vi "Control.vi"() -> ()   [LabVIEW 2012]
uses:
  <vilib>/express/express analysis/Spectral/Block/exnSpectralBlock spectral measurements peak poly.vi
  <vilib>/express/express analysis/Spectral/Block/exnSpectralBlock spectral measurements peak DDT.vi
  <vilib>/express/express analysis/Spectral/XNode/ExpressSpectralMeasurementsBlockNode.xnode
  <vilib>/Analysis/NI_AALPro.lvlib
panel:
  out "Waveform Graph":dynamicdata(graph)
  out "GrabO 5":dbl[](array[numeric])
  out "GrabO 4":dbl[](array[numeric])
  out "In Range?":bool[](array[boolean])
  out "Entrada":dbl[](array[numeric])
  out "GrabO 3":dbl[](array[numeric])
  out "GrabO 2":dbl[](array[numeric])
  out "GrabO":dbl[](array[numeric])
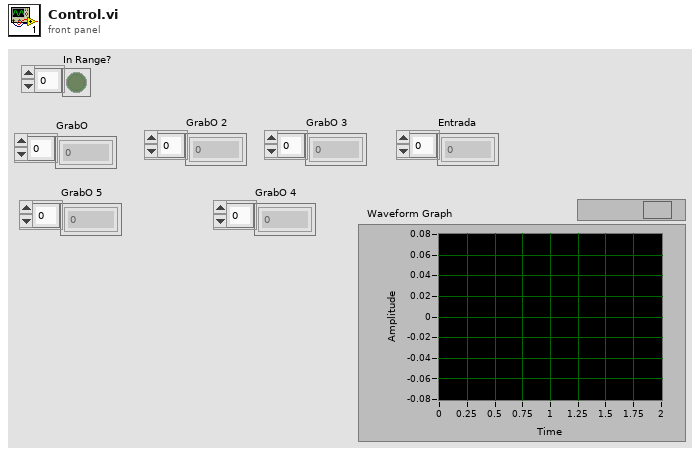
[diagram p1: front panel]
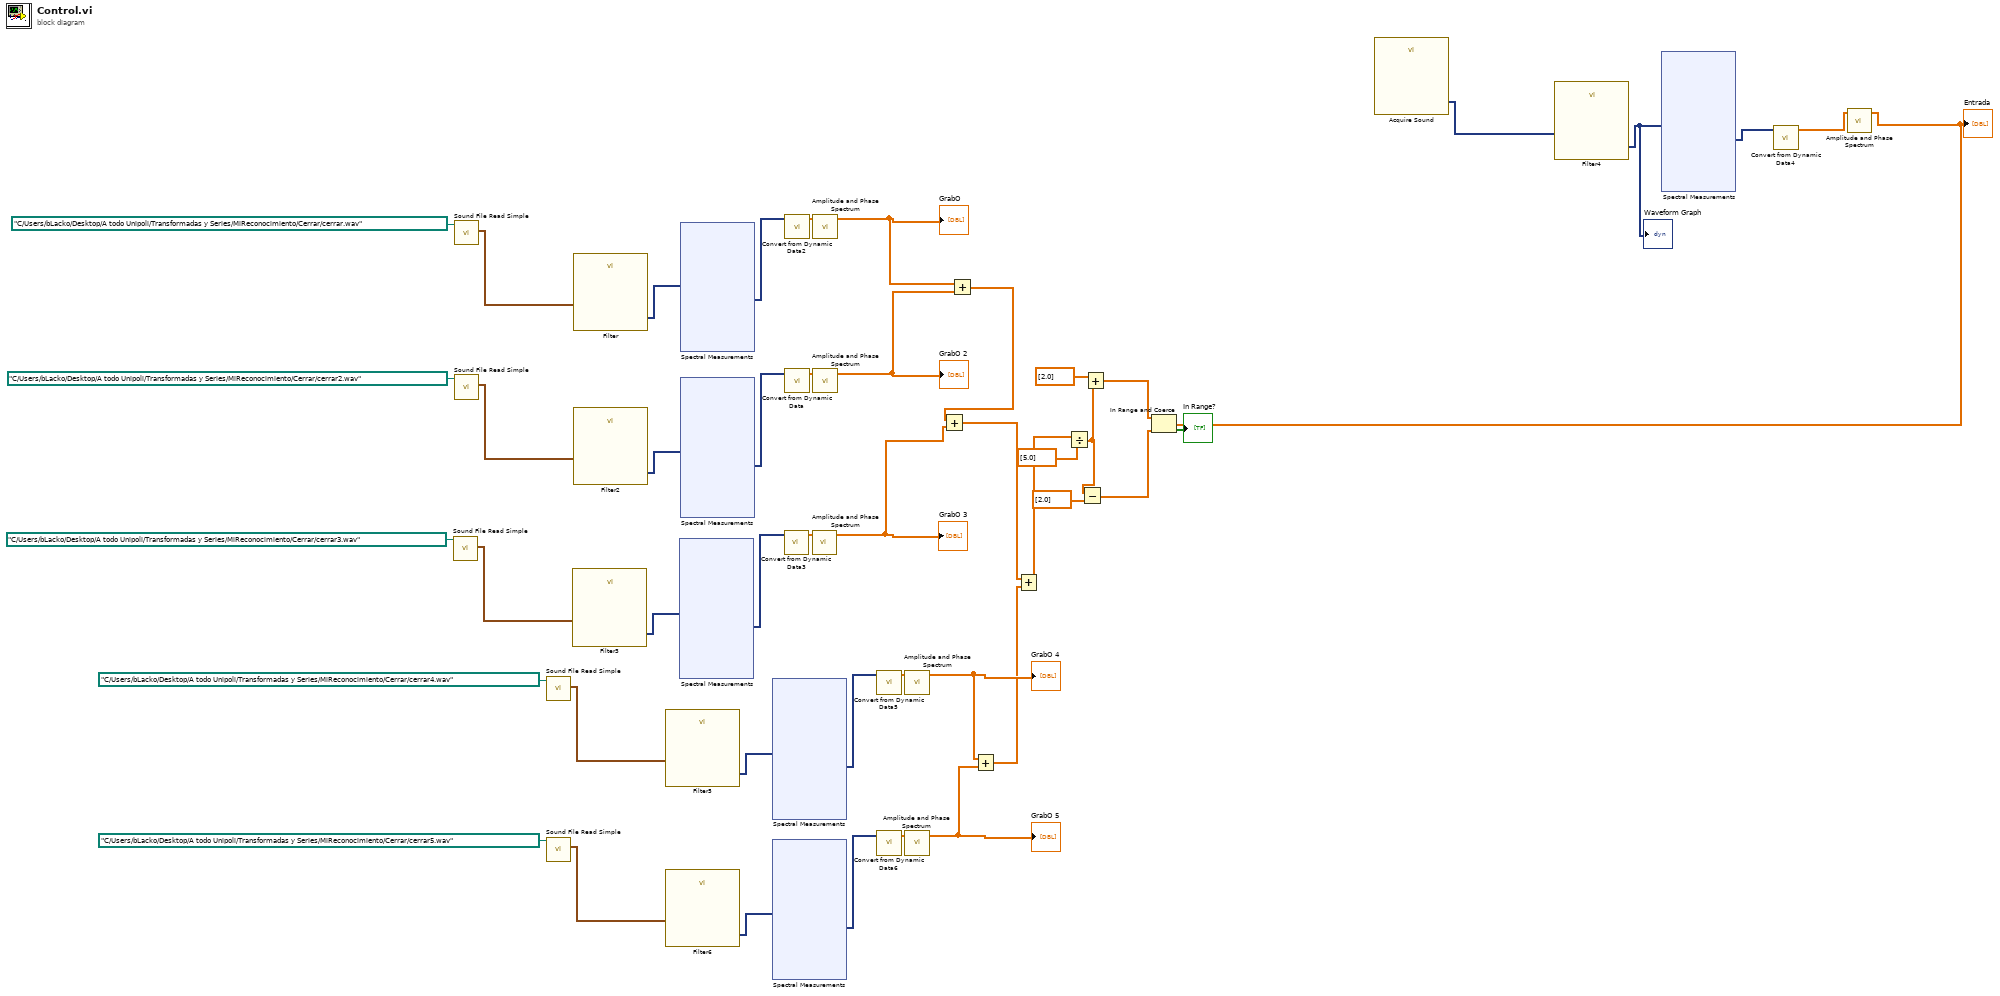
[diagram p0: block diagram]
diagram:
  n1 = call <vilib>:"Sound File Read Simple.vi"("path"=path "C:/Users/bLacko/Desktop/A todo Unipoli/Transformadas y Series/MiReconocimiento/Cerrar/cerrar3.wav") -> ("data"=w39:waveform(dbl)[])  [unwired: 7 in, 3 out]
  n2 = call <vilib>:"Sound File Read Simple.vi"("path"=path "C:/Users/bLacko/Desktop/A todo Unipoli/Transformadas y Series/MiReconocimiento/Cerrar/cerrar.wav") -> ("data"=w45:waveform(dbl)[])  [unwired: 7 in, 3 out]
  n3 = call <vilib>:"Sound File Read Simple.vi"("path"=path "C:/Users/bLacko/Desktop/A todo Unipoli/Transformadas y Series/MiReconocimiento/Cerrar/cerrar2.wav") -> ("data"=w42:waveform(dbl)[])  [unwired: 7 in, 3 out]
  n4 = call <vilib>:"Sound File Read Simple.vi"("path"=path "C:/Users/bLacko/Desktop/A todo Unipoli/Transformadas y Series/MiReconocimiento/Cerrar/cerrar4.wav") -> ("data"=w21:waveform(dbl)[])  [unwired: 7 in, 3 out]
  n5 = call <vilib>:"Sound File Read Simple.vi"("path"=path "C:/Users/bLacko/Desktop/A todo Unipoli/Transformadas y Series/MiReconocimiento/Cerrar/cerrar5.wav") -> ("data"=w17:waveform(dbl)[])  [unwired: 7 in, 3 out]
  n6 = call "Filter3"("Signal"=w39) -> ("Filtered Signal"=w4:dynamicdata)  [unwired: 9 in, 1 out]
  n7 = call "Filter"("Signal"=w45) -> ("Filtered Signal"=w6:dynamicdata)  [unwired: 9 in, 1 out]
  n8 = call "Filter2"("Signal"=w42) -> ("Filtered Signal"=w5:dynamicdata)  [unwired: 9 in, 1 out]
  n9 = call "Filter5"("Signal"=w21) -> ("Filtered Signal"=w3:dynamicdata)  [unwired: 9 in, 1 out]
  n10 = call "Filter6"("Signal"=w17) -> ("Filtered Signal"=w2:dynamicdata)  [unwired: 9 in, 1 out]
  n11 = xnode "Spectral Measurements"("Signals"=w4) -> ("FFT - (Peak)"=w38:dynamicdata)  [unwired: 1 in, 2 out]
  n12 = xnode "Spectral Measurements"("Signals"=w6) -> ("FFT - (Peak)"=w44:dynamicdata)  [unwired: 1 in, 2 out]
  n13 = xnode "Spectral Measurements"("Signals"=w5) -> ("FFT - (Peak)"=w41:dynamicdata)  [unwired: 1 in, 2 out]
  n14 = xnode "Spectral Measurements"("Signals"=w3) -> ("FFT - (Peak)"=w20:dynamicdata)  [unwired: 1 in, 2 out]
  n15 = xnode "Spectral Measurements"("Signals"=w2) -> ("FFT - (Peak)"=w16:dynamicdata)  [unwired: 1 in, 2 out]
  n16 = call "Convert from Dynamic Data3"("Dynamic Data Type"=w38) -> ("Array"=w37:dbl[])  [unwired: 3 in]
  n17 = call "Convert from Dynamic Data2"("Dynamic Data Type"=w44) -> ("Array"=w43:dbl[])  [unwired: 3 in]
  n18 = call "Convert from Dynamic Data"("Dynamic Data Type"=w41) -> ("Array"=w40:dbl[])  [unwired: 3 in]
  n19 = call <vilib>:"Amplitude and Phase Spectrum.vi"("Signal (V)"=w37) -> ("Amp Spectrum Mag (Vrms)"=w11:dbl[])  [unwired: 2 in, 2 out]
  "GrabO 3" <- w11
  n20 = call <vilib>:"Amplitude and Phase Spectrum.vi"("Signal (V)"=w43) -> ("Amp Spectrum Mag (Vrms)"=w31:dbl[])  [unwired: 2 in, 2 out]
  "GrabO" <- w31
  n21 = call <vilib>:"Amplitude and Phase Spectrum.vi"("Signal (V)"=w40) -> ("Amp Spectrum Mag (Vrms)"=w30:dbl[])  [unwired: 2 in, 2 out]
  "GrabO 2" <- w30
  n22 = call "Convert from Dynamic Data5"("Dynamic Data Type"=w20) -> ("Array"=w19:dbl[])  [unwired: 3 in]
  n23 = call "Convert from Dynamic Data6"("Dynamic Data Type"=w16) -> ("Array"=w15:dbl[])  [unwired: 3 in]
  n24 = call <vilib>:"Amplitude and Phase Spectrum.vi"("Signal (V)"=w19) -> ("Amp Spectrum Mag (Vrms)"=w13:dbl[])  [unwired: 2 in, 2 out]
  "GrabO 4" <- w13
  n25 = call <vilib>:"Amplitude and Phase Spectrum.vi"("Signal (V)"=w15) -> ("Amp Spectrum Mag (Vrms)"=w12:dbl[])  [unwired: 2 in, 2 out]
  "GrabO 5" <- w12
  n26 = Add(x=w31, y=w30) -> (x+y=w10:dbl[])
  n27 = Add(x=w10, y=w11) -> (x+y=w8:dbl[])
  n28 = Add(x=w13, y=w12) -> (x+y=w9:dbl[])
  n29 = Add(x=w8, y=w9) -> (x+y=w7:dbl[])
  n30 = Divide(x=w7, y=dbl[] [5.0]) -> (x/y=w28:dbl[])
  n31 = Subtract(x=w28, y=dbl[] [2.0]) -> (x-y=w24:dbl[])
  n32 = Add(x=dbl[] [2.0], y=w28) -> (x+y=w25:dbl[])
  n33 = call "Acquire Sound"() -> ("Data"=w36:dynamicdata)  [unwired: 18 in, 1 out]
  n34 = call "Filter4"("Signal"=w36) -> ("Filtered Signal"=w1:dynamicdata)  [unwired: 9 in, 1 out]
  "Waveform Graph" <- w1
  n35 = xnode "Spectral Measurements"("Signals"=w1) -> ("FFT - (Peak)"=w35:dynamicdata)  [unwired: 1 in, 2 out]
  n36 = call "Convert from Dynamic Data4"("Dynamic Data Type"=w35) -> ("Array"=w34:dbl[])  [unwired: 3 in]
  n37 = call <vilib>:"Amplitude and Phase Spectrum.vi"("Signal (V)"=w34) -> ("Amp Spectrum Mag (Vrms)"=w23:dbl[])  [unwired: 2 in, 2 out]
  "Entrada" <- w23
  n38 = In Range and Coerce(upper limit=w25, x=w23, lower limit=w24) -> (In Range?=→"In Range?":bool[])  [unwired: 1 out]
